vi "black_key_width.vi"(10 "C# or D#?":bool, 11 "midi-ui in":refnum<class "midi-ui.lvclass">) -> (2 "Black Key Width":dbl, 3 "midi-ui out":refnum<class "midi-ui.lvclass">)   [LabVIEW 2020, in "midi-ui.lvclass"]
uses:
  midi-ui.lvclass
  midi-ui.lvclass/midi-ui.ctl
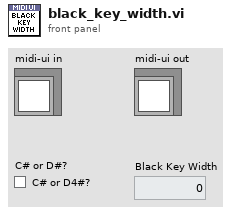
[diagram p1: front panel]
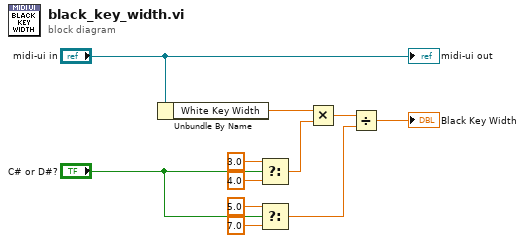
[diagram p0: block diagram]
diagram:
  n1 = Unbundle By Name("midi-ui in") -> ("White Key Width"=w10:dbl)
  n2 = Select(t=3.0, s="C# or D#?", f=4.0) -> (s? t:f=w7:dbl)
  n3 = Select(t=5.0, s="C# or D#?", f=7.0) -> (s? t:f=w6:dbl)
  n4 = Multiply(x=w10, y=w7) -> (x*y=w9:dbl)
  n5 = Divide(x=w9, y=w6) -> (x/y=→"Black Key Width":dbl)
  "midi-ui out" <- "midi-ui in"
